vi "Write SCH Config Parameters.vi"(6 "key":string, 7 "section":string, 8 "error in (no error)":errorcluster, 9 "FPGA Configuration Values":T1={"Ln2 Filter Size"=10, "VT Quench Tick Limit"=4000000, "VT Quench Volt Limit"=0.1999969482421875, "Joint Tick Limit"=4000000, "Joint Volt Limit"=9.98377799987793e-07, "CoWound Volt Limit"=0.20001220703125, "CoWound Tick Limit"=4000000, "SC Bus Limit"=0.001953125, "SC Bus Tick Limit"=4000000, "ResMag Tick Limit"=1000000, "DAQ Cycle Ticks"=4096, "Res Mag dI/dt Delay"=256, "dI/dT scaling"=38.14697265625, "Pressure Inlet Limit (BarA)"=6.0, "Bore Tube Volt Limit"=0.5999999940395355, "Pressure Outlet Limit (BarA)"=5.0, "Activation Current (kA)"=0.5, "Dump Resistor Scale Factor"=200.0, "Co-Wound Asymmetry Factor"=0.0, "Co-Wound Scale Factor"=200.0, "Layer Scale Factors"=[3.0, 3.0, 3.0, 3.0, 3.0, 3.0, 3.0, 3.0, 3.0, 3.0, 3.0, 3.0, 3.0, 3.0, 3.0, 3.0, 3.0, 3.0], "Fudge Factors"=[0.0, 0.0, 0.0, 0.0, 0.0, 0.0, 0.0, 0.0, 0.0, 0.0, 0.0, 0.0, 0.0, 0.0, 0.0, 0.0], "Joint Scale Factors"=[1.0013580322265625e-05, 1.0013580322265625e-05, 1.0013580322265625e-05, 1.0013580322265625e-05, 1.0013580322265625e-05, 1.0013580322265625e-05, 1.0013580322265625e-05, 1.0013580322265625e-05], "SC Bus Scale"=[0.0009765326976776123, 0.0009765326976776123, 0.0009765326976776123, 0.0009765326976776123, 0.0009765326976776123, 0.0009765326976776123], "Pressure Scale Factor"=[1.723690003156662, 1.723690003156662, 1.723690003156662, 1.723690003156662], "# Consecutive Zeros Fault"=1000, "Digitize Convert Ticks"=200, "Digitize Reset Ticks"=400, "Convert Clock Ticks"=20, "Digitize Read Delay Ticks"=13, "Digitize # Bits"=16, "HTS Lead Tick Limit"=4000000, "Res Lead Tick Limit"=4000000, "HTS Lead Trip"=0.20000000298023224, "Res Lead Limit"=0.001953125, "HTS Lead FRZ"=0.006999999284744263, "HTS Lead Warn"=0.0010000020265579224, "Low Current (kA)"=0.04500000178814, "Low Current Ticks"=400000000, "Low Current Delay Factor"=100, "HTS Resistance (nOhm)"=[0.0, 0.0], "Ticks to Close Relief"=80000000, "All Breaker Tick Limit"=400000000, "HTS Offset (microV)"=[0.0, 0.0], "Delay Ticks Between Bkr Reset"=1200000000, "Breaker Reset Ticks"=400000000, "PS Enable Reset Ticks"=400000000, "Reset Digitizer Ticks"=400000000} {"HTS Offset (microV)" format="%_6g"; "HTS Resistance (nOhm)" format="%_6g"; "HTS Lead Warn" format="%_6g"; "HTS Lead FRZ" format="%_6g"; "Res Lead Limit" format="%_6g"; "HTS Lead Trip" format="%_6g"; "Pressure Scale Factor" format="%_6g"; "Joint Scale Factors" format="%_6g"; "Fudge Factors" format="%.7g"; "Co-Wound Asymmetry Factor" format="%.8g"; "Activation Current (kA)" format="%_6g"; "Pressure Outlet Limit (BarA)" format="%.5g"; "Bore Tube Volt Limit" format="%_6g"; "Pressure Inlet Limit (BarA)" format="%.5g"; "dI/dT scaling" format="%.11g"; "SC Bus Limit" format="%_6g"; "Joint Volt Limit" format="%_6g"; "VT Quench Volt Limit" format="%.5g"}, 10 "refnum in":T2) -> (0 "error out":errorcluster, 2 "refnum out":T2)   [LabVIEW 2018]
doc: "Author: Scott Hannahs <sth@magnet.fsu.edu>\nCopyright 2018 Florida State University, All rights reserved."
uses:
  <vilib>/Utility/config.llb/Config Data RefNum.ctl
  SCH Data Controls/FPGA Configure Parameters.ctl
  <vilib>/Utility/config.llb/Write Key (String).vi
  <vilib>/Utility/config.llb/NI_LVConfig.lvlib
panel:
  out "string out":string
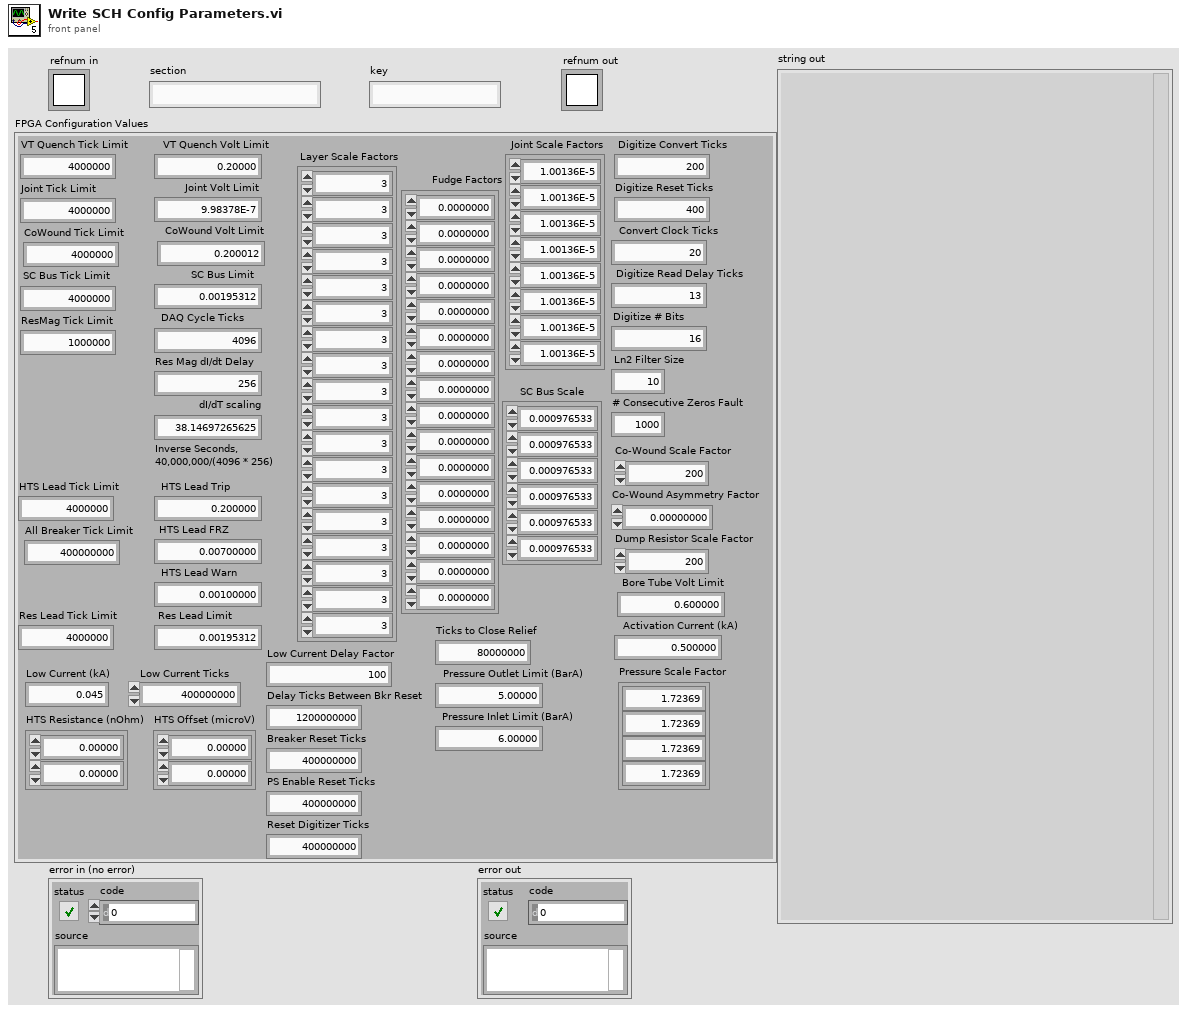
[diagram p1: front panel]
types:
  T1 = typedef "FPGA Configure Parameters.ctl" = cluster{"Ln2 Filter Size":i16, "VT Quench Tick Limit":u32, "VT Quench Volt Limit":dbl, "Joint Tick Limit":u32, "Joint Volt Limit":dbl, "CoWound Volt Limit":dbl, "CoWound Tick Limit":u32, "SC Bus Limit":dbl, "SC Bus Tick Limit":u32, "ResMag Tick Limit":u32, "DAQ Cycle Ticks":u32, "Res Mag dI/dt Delay":u32, "dI/dT scaling":dbl, "Pressure Inlet Limit (BarA)":dbl, "Bore Tube Volt Limit":dbl, "Pressure Outlet Limit (BarA)":dbl, "Activation Current (kA)":dbl, "Dump Resistor Scale Factor":dbl, "Co-Wound Asymmetry Factor":dbl, "Co-Wound Scale Factor":dbl, "Layer Scale Factors":dbl[], "Fudge Factors":dbl[], "Joint Scale Factors":dbl[], "SC Bus Scale":dbl[], "Pressure Scale Factor":dbl[], "# Consecutive Zeros Fault":i16, "Digitize Convert Ticks":u32, "Digitize Reset Ticks":u32, "Convert Clock Ticks":u32, "Digitize Read Delay Ticks":u32, "Digitize # Bits":u32, "HTS Lead Tick Limit":u32, "Res Lead Tick Limit":u32, "HTS Lead Trip":dbl, "Res Lead Limit":dbl, "HTS Lead FRZ":dbl, "HTS Lead Warn":dbl, "Low Current (kA)":dbl, "Low Current Ticks":u32, "Low Current Delay Factor":u16, "HTS Resistance (nOhm)":dbl[], "Ticks to Close Relief":u32, "All Breaker Tick Limit":u32, "HTS Offset (microV)":dbl[], "Delay Ticks Between Bkr Reset":u32, "Breaker Reset Ticks":u32, "PS Enable Reset Ticks":u32, "Reset Digitizer Ticks":u32}
  T2 = typedef "NI_LVConfig.lvlib/Config Data RefNum.ctl" = refnum<k1>
  T3 = enum16{"Native", "Native Command Line", "UNIX", "Macintosh", "DOS"}
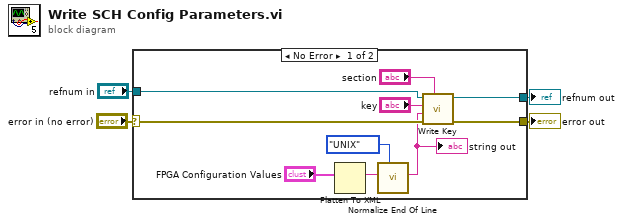
[diagram p0: block diagram]
diagram:
  n1 = case shown="No Error" "error in (no error)" {
    selector: "error in (no error)" -> [w7 w16]
    tunnel: [w10 w16] -> w3
    tunnel: "refnum in" -> [w9 w15]
    tunnel: [w8 w15] -> w1
    frame No Error {
      n2 = Flatten To XML(anything="FPGA Configuration Values") -> (xml string=w13:string)
      n3 = call <vilib>:"Normalize End Of Line.vi"("end of line (Native)"=T3."UNIX", "string in"=w13) -> ("string out"=w6:string)  [unwired: 6 in]
      "string out" <- w6
      n4 = call-poly <vilib>:"Write Key.vi"("section"="section", "error in (no error)"=w7, "value"=w6, "key"="key", "refnum"=w9) -> ("error out"=w10:errorcluster, "refnum out"=w8:T2)  [unwired: 4 in, 1 out]
    }
    frame Error {
    }
  }
  "error out" <- w3
  "refnum out" <- w1
